vi "insert into came from.vi"(9 "Node came from":cluster{"Weight":dbl, "Row":dbl, "Col":dbl}, 10 "Node":cluster{"Weight":dbl, "Row":dbl, "Col":dbl}, 11 "Came_from":T1(array[cluster])) -> (3 "Came_from out":T1(array[cluster]))   [LabVIEW 2014]
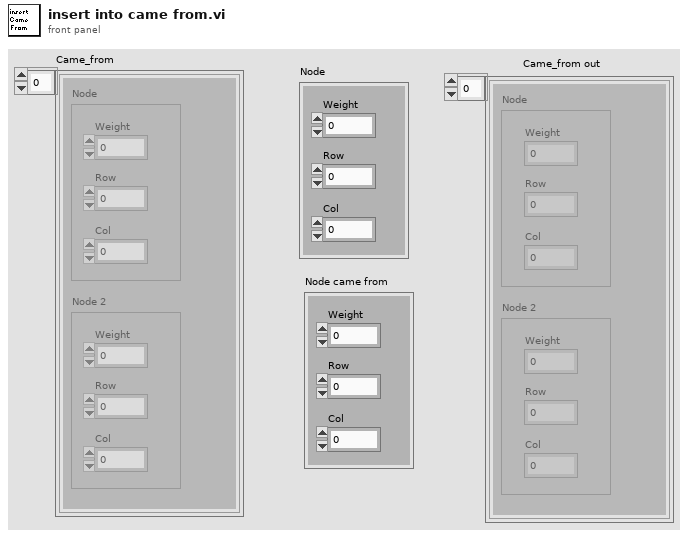
[diagram p1: front panel]
types:
  T1 = cluster{"Node":cluster{"Weight":dbl, "Row":dbl, "Col":dbl}, "Node 2":cluster{"Weight":dbl, "Row":dbl, "Col":dbl}}[]
  T2 = cluster{"Node":cluster{"Weight":dbl, "Row":dbl, "Col":dbl}, "Node 2":cluster{"Weight":dbl, "Row":dbl, "Col":dbl}}
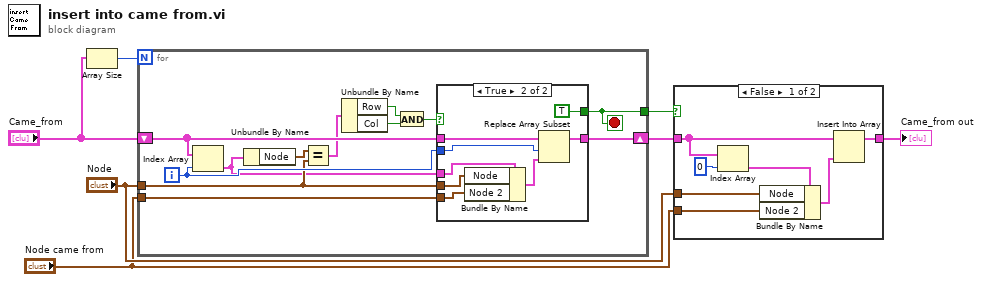
[diagram p0: block diagram]
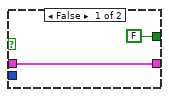
[diagram p3: hidden frame]
diagram:
  n1 = Array Size(array="Came_from") -> (size(s)=w7:i32)
  n2 = for {
    N: w7 -> [_]
    tunnel: "Node" -> [w16]
    tunnel: "Node came from" -> [w17]
    shift-right: [w13] -> w4
    shift-left: "Came_from" -> [w14]
    tunnel: [w12] -> w5
    i -> [w18]
    stop <- w12 stop-if-true
    n3 = Index Array(array=w14, index=w18) -> (element=w15:T2)
    n4 = Unbundle By Name(w15) -> ("Node"=w19:cluster{"Weight":dbl, "Row":dbl, "Col":dbl})
    n5 = Equal?(x=w19, y=w16) -> (x = y?=w11:cluster{"Weight":bool, "Row":bool, "Col":bool})
    n6 = Unbundle By Name(w11) -> ("Row"=w10:bool, "Col"=w9:bool)
    n7 = And(x=w10, y=w9) -> (x .and. y?=w8:bool)
    n8 = case shown="True" w8 {
      tunnel: w18 -> [_ w25]
      tunnel: w17 -> [_ w27]
      tunnel: w16 -> [_ w28]
      tunnel: w15 -> [_ w29]
      tunnel: w14 -> [w20 w26]
      tunnel: [w20 w23] -> w13
      tunnel: [FALSE TRUE] -> w12
      frame False {
      }
      frame True {
        n9 = Bundle By Name(cluster=w29, "Node"=w28, "Node 2"=w27) -> (w24:T2)
        n10 = Replace Array Subset(array=w26, new element=w24, index=w25) -> (w23:T1)
      }
    }
  }
  n11 = case shown="False" w5 {
    tunnel: w4 -> [w36 w37]
    tunnel: "Node" -> [w33 _]
    tunnel: "Node came from" -> [w32 _]
    tunnel: [w30 w37] -> w1
    frame False {
      n12 = Index Array(array=w36, index=0) -> (element=w34:T2)
      n13 = Bundle By Name(cluster=w34, "Node"=w33, "Node 2"=w32) -> (w31:T2)
      n14 = Insert Into Array(array=w36, new element=w31) -> (w30:T1)  [unwired: 1 in]
    }
    frame True {
    }
  }
  "Came_from out" <- w1
